vi "Telescope GUI.vi"(9 "Standalone":bool=TRUE, 10 "Init Data":variant, 11 "Telescope Name":string) -> ()   [LabVIEW 2024]
uses:
  typedefs/CC enum Operation Mode.ctl
  Telescope cluster Settings.ctl
  CC cluster Telescope Offsets.ctl
  typedefs/CC cluster sidereal rate.ctl
  Telescope cluster Equinox.ctl
  Telescope cluster Parallax.ctl
  Telescope cluster Rotator.ctl
  Telesope ring Frame.ctl
  Subsystems/SS typedef cluster Instrument Command Queue Data.ctl
  Subsystems/SS cluster Data Queue type.ctl
  Telescope.lvclass
  Telescope cluster Status.ctl
  typedefs/CC cluster RA and DEC.ctl
  Telescope enum Status.ctl
  hk-channel-class/hk-channel-class/HK Item/HK Item.lvclass
  typedefs/CC cluster Object.ctl
  typedefs/cc cluster muRA muDEC.ctl
  typedefs/CC cluster Alarm Data.ctl
  hk-channel-class/hk-channel-class/HK Item/HK Channel cluster Telemetry Data.ctl
  hk-channel-class/hk-channel-class/HK Item/HK Channel enum Data Type.ctl
  hk-channel-class/hk-channel-class/HK Item/HK Item.lvclass/HK Item.ctl
  hk-channel-class/hk-channel-class/HK Alarms/HK Alarm enum Status.ctl
panel:
  in  "Mode":T1
  in  "Tab Control":T2(tab)
  in  "Tab Control 2":T3(tab)
  in  "Target Settings":T4={"RA Proper Motion"=0.0, "DEC Proper Motion"=0.0, "Equinox"=2000.0}
  in  "Wavelength":dbl=1.67
  in  "Frac Rate":dbl=1.0
  in  "Frame":T5=enum."FK5"
  in  "Equinox":T6={"Equinox Year"=2000, "Equinox Prefix"="J"}
  in  "Diff Track":T7
  in  "Parallax":T8
  in  "Rotator":T9={"Frame"="Target", "PA"=0.0}
  in  "Offsets":T10 caption="Offsets (arcSec)"
  in  "Target  DEC Deg":dbl
  in  "Target  RA Deg":dbl
  in  "Target DEC":string
  in  "Target RA":string
  out "DEC Str":string
  out "RA str":string
  out "Moving":bool
  out "Focus Position":dbl format="%.3g"
  out "DEC":dbl
  out "RA":dbl
  out "Telescope Time":timestamp
  out "Connected":bool
  in  "Home Button":bool
  in  "Stop Button":bool
  in  "Move To":bool
  in  "Focus Home":bool
  in  "Move Focus":bool
  in  "Position":dbl format="%.3g"
  in  "Debug":bool
  in  "Reconnect":bool
  in  "Settings Button":bool
  out "Response":string
  in  "Telescope Type":u16(ring) items=["Simulation", "Lowell", "PRIME"]
  out "Messages":string
  out "Cmd Sent":string
  in  "Close":bool
  out "Connect Message":string
  in  "Housekeeping Data":i32(listbox)
  # "Status"
  # "Focus"
  # "HH:MM:SS.s"
  # "Degrees"
  # "HH:MM:SS.s"
  # "Degrees"
  # "microns"
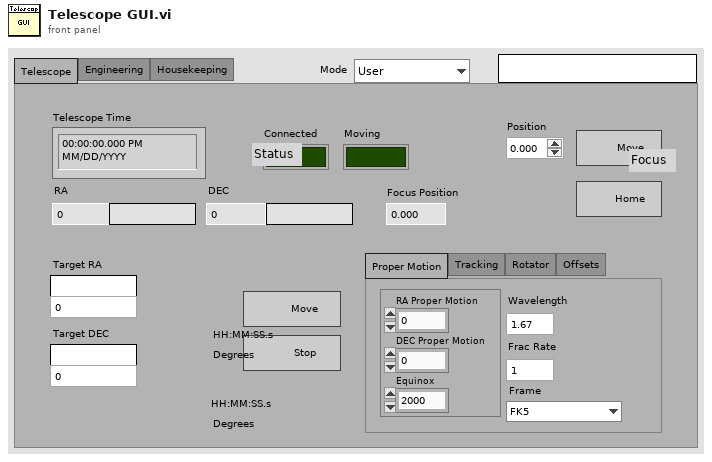
[diagram p1: front panel]
types:
  T1 = typedef "CC enum Operation Mode.ctl" = enum16{"User", "Engineering"}
  T2 = enum32{"Telescope", "Engineering", "Housekeeping"}
  T3 = enum32{"Proper Motion", "Tracking", "Rotator", "Offsets"}
  T4 = typedef "Telescope cluster Settings.ctl" = cluster{"RA Proper Motion":dbl, "DEC Proper Motion":dbl, "Equinox":dbl}
  T5 = typedef "Telesope ring Frame.ctl" = enum16{"FK4", "FK5", "APPT", "GAPPT", "AZEL"}
  T6 = typedef "Telescope cluster Equinox.ctl" = cluster{"Equinox Year":i32, "Equinox Prefix":string}
  T7 = typedef "CC cluster sidereal rate.ctl" = cluster{"dRA":dbl, "dDEC":dbl}
  T8 = typedef "Telescope cluster Parallax.ctl" = cluster{"Parallax":dbl, "rv kps":dbl}
  T9 = typedef "Telescope cluster Rotator.ctl" = cluster{"Frame":string, "PA":dbl}
  T10 = typedef "CC cluster Telescope Offsets.ctl" = cluster{"RA":dbl, "DEC":dbl, "ROT":dbl}
  T11 = typedef "SS typedef cluster Instrument Command Queue Data.ctl" = cluster{"Cmd":string, "Parameters":variant}
  T12 = typedef "Telescope.lvclass/Telescope cluster Status.ctl" = cluster{"Position":T13, "Connected":bool, "Status":T14, "Curr Time":timestamp, "Status Word":u32, "Focus Pos A":dbl, "UTC Time":timestamp, "Local Sidreal Time":dbl, "Azimuth":dbl, "Altitude":dbl, "Rotator Angle":dbl, "RA String":string, "DEC String":string, "secZ":dbl, "Focus Pos B":dbl, "Focus Pos A-B":dbl, "Rotator Offset":dbl, "Time Offset":dbl, "Dome Angle":dbl, "Dome Status Word":u32, "Dome Moving":bool}
  T13 = typedef "CC cluster RA and DEC.ctl" = cluster{"RA":dbl, "DEC":dbl}
  T14 = typedef "Telescope.lvclass/Telescope enum Status.ctl" = enum16{"Initializing", "Ready", "Moving", "Focusing", "Error"}
  T15 = typedef "CC cluster Object.ctl" = cluster{"Object":cluster{"Name":string}, "Sidereal Rate":T7, "RA and DEC":T13, "Proper Motion":T16, "Offsets":T10, "Equinox":T6, "Parallax":T8, "Rotator":T9, "Frame":T5, "Frac Rate":dbl, "Wavelength":dbl}
  T16 = typedef "cc cluster muRA muDEC.ctl" = cluster{"muRA":dbl, "muDEC":dbl, "Epoch":dbl}
  T17 = cluster{"state":refnum<user-event>, "cmd q":refnum<queue>, "Cmd":T11, "Data Q":refnum<queue>, "error":errorcluster, "next poll":timestamp, "Telescope":refnum<class "Telescope.lvclass">, "Telescope Name":string, "poll":bool, "Telescope Status":T12, "Channel List":refnum<class "HK Item.lvclass">[], "Focus Pos":dbl, "Move Position":T15}
  T18 = typedef "CC cluster Alarm Data.ctl" = cluster{"Measured Value":dbl, "Alarm Low":dbl, "Alarm High":dbl, "Message":string, "Source":string}
  T19 = typedef "SS cluster Data Queue type.ctl" = cluster{"Source":string, "Type":string, "Data":variant}
  T20 = enum32{"Page Enabled", "Page Disabled", "Page Disabled & Grayed"}
  T21 = typedef "HK Item.lvclass/HK Channel enum Data Type.ctl" = enum16{"Floating Point", "Integer", "Enum", "String", "Waveform", "File"}
  T22 = typedef "HK Item.lvclass/HK Channel cluster Telemetry Data.ctl" = cluster{"Ch Names":string[], "Ch Values":dbl[], "Timestamp":timestamp, "Data Type":T21}
  T23 = typedef "CC cluster Device Index.ctl" = cluster{"Device Type Name":string, "Curr Device Name":string, "All Instances":string[]}
  T24 = typedef "HK Item.lvclass/HK Channel Units and Setup.ctl" = cluster{"Unit Type":string, "Units":string, "Configuration":string, "Digits":i32, "Data Type":T21, "Exponential?":bool, "Source":string}
  T25 = typedef "HK Item.lvclass/HK Alarm enum Status.ctl" = enum16{"No Alarm", "Red Low", "Red High", "Yellow Low", "Yellow High"}
  T26 = enum32{"invalid app kind", "Development System", "Run Time System", "Student Edition", "Embedded LabVIEW", "Evaluation", "Custom"}
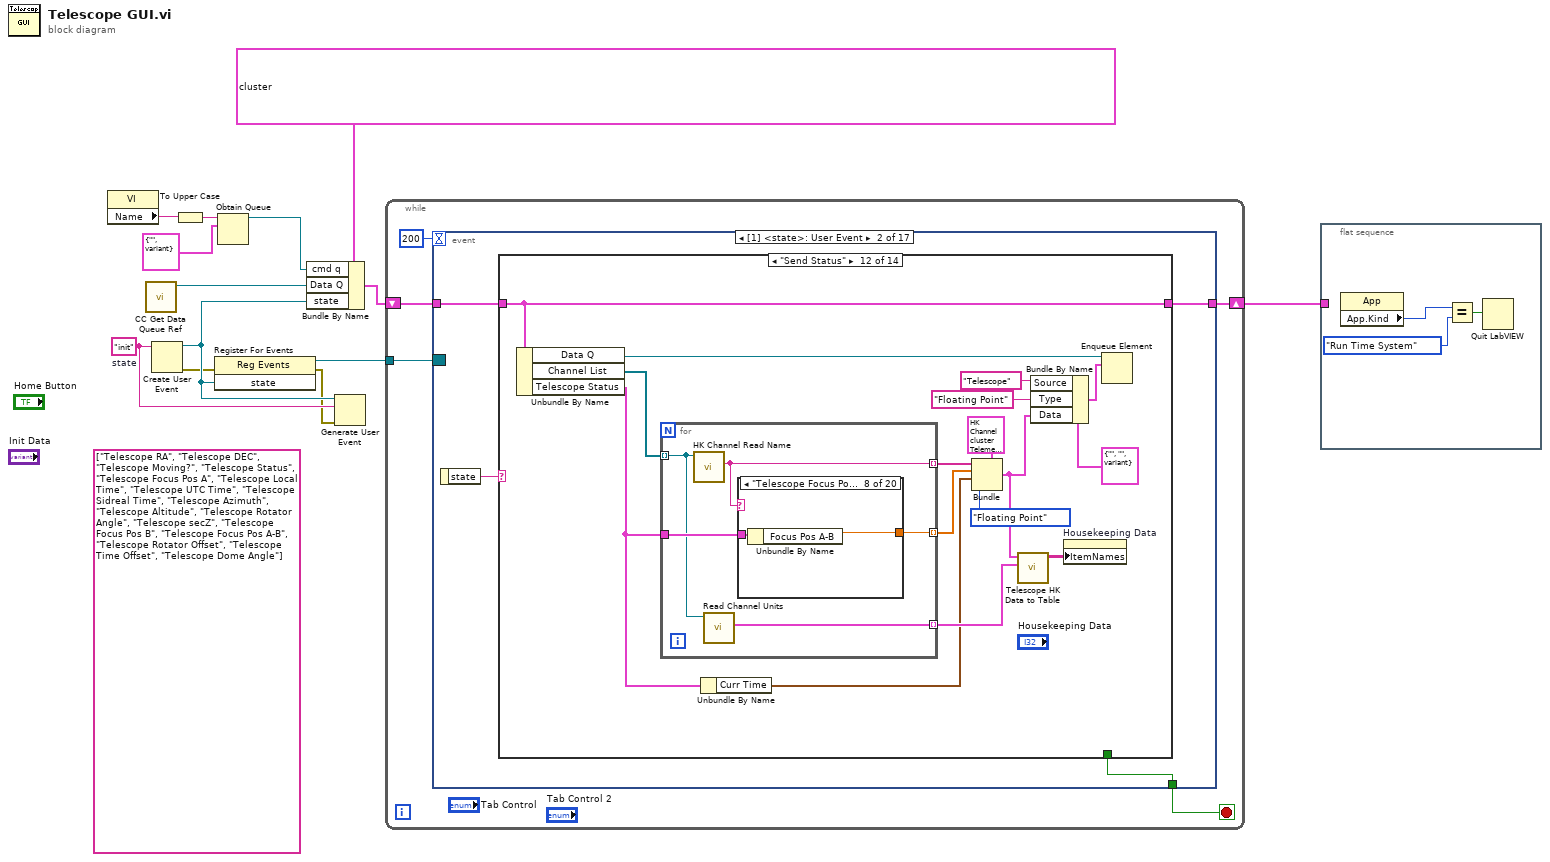
[diagram p0: block diagram]
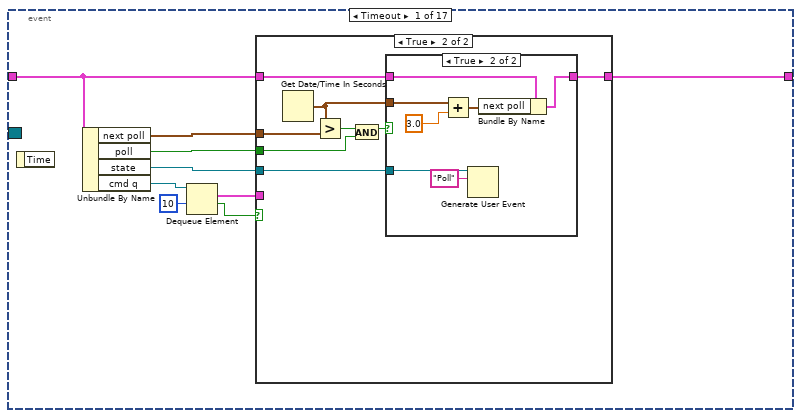
[diagram p2: hidden frame]
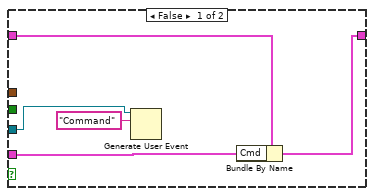
[diagram p3: hidden frame]
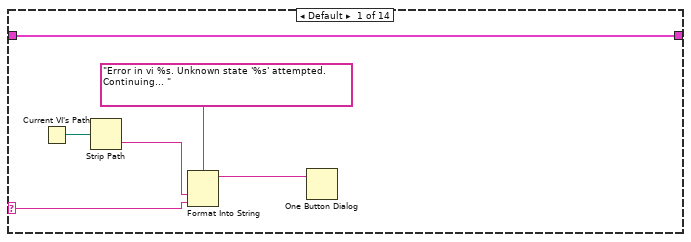
[diagram p5: hidden frame]
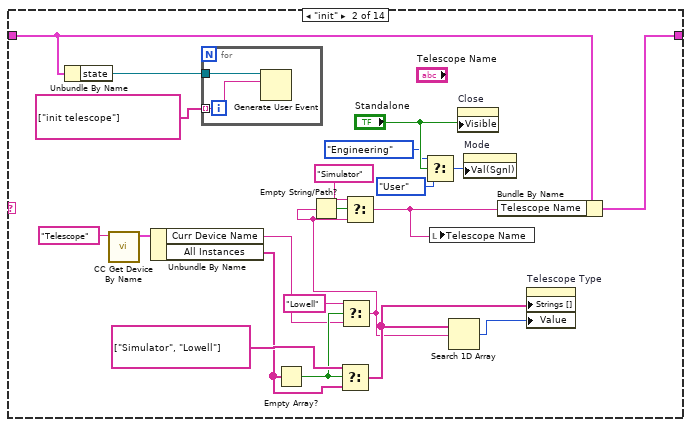
[diagram p6: hidden frame]
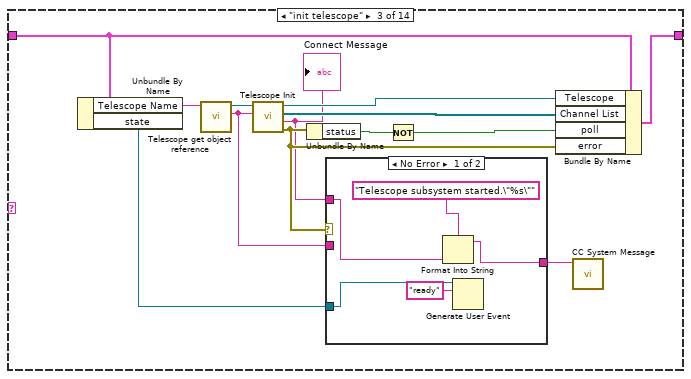
[diagram p7: hidden frame]
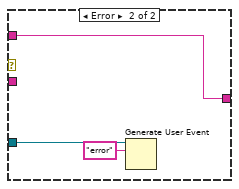
[diagram p8: hidden frame]
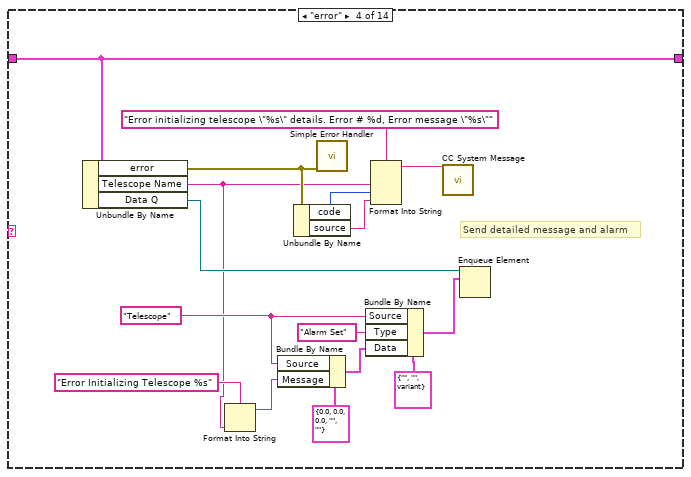
[diagram p9: hidden frame]
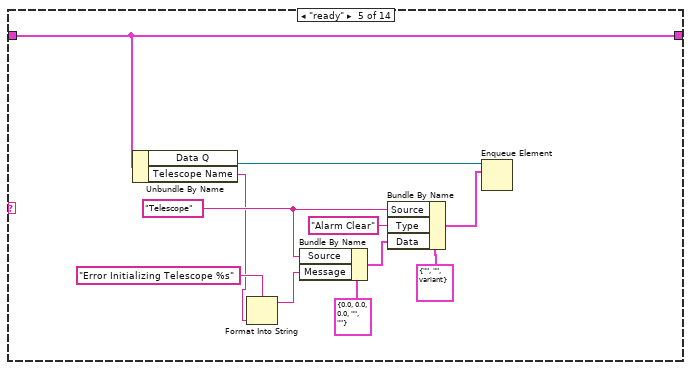
[diagram p10: hidden frame]
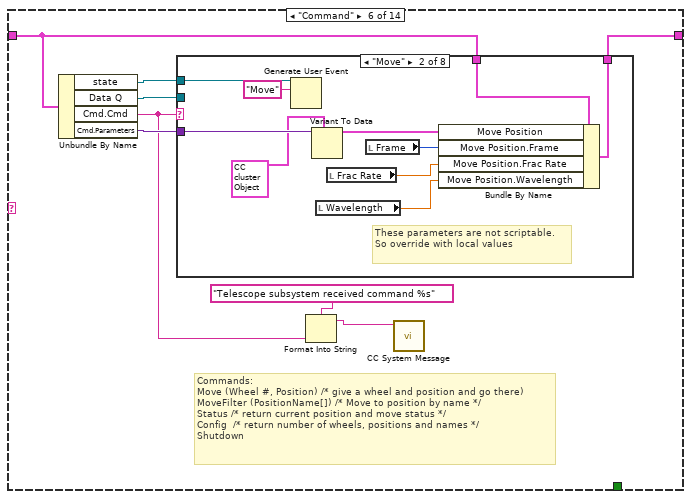
[diagram p11: hidden frame]
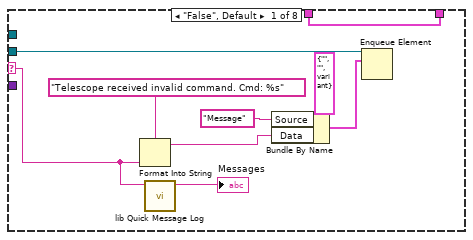
[diagram p12: hidden frame]
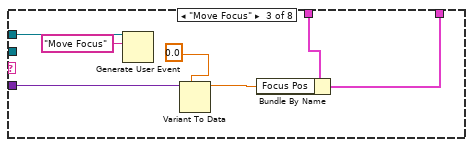
[diagram p13: hidden frame]
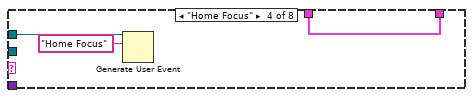
[diagram p14: hidden frame]
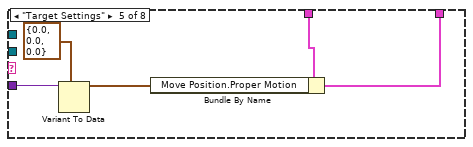
[diagram p15: hidden frame]
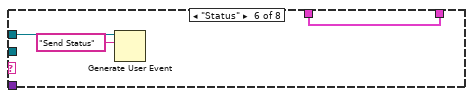
[diagram p16: hidden frame]
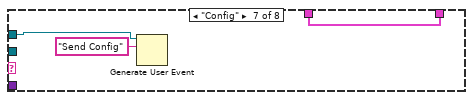
[diagram p17: hidden frame]
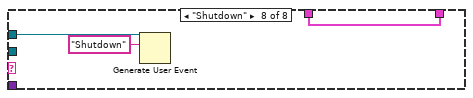
[diagram p18: hidden frame]
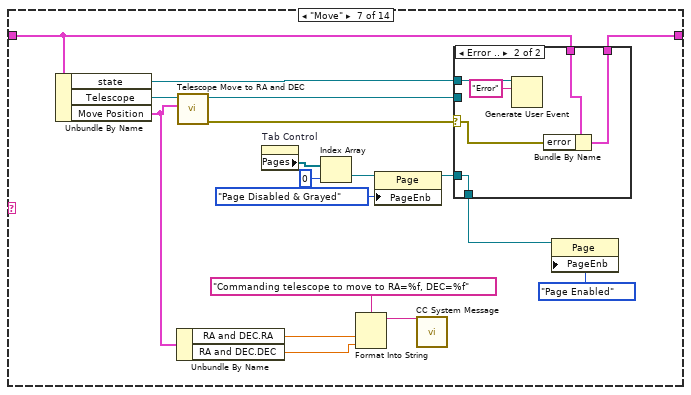
[diagram p19: hidden frame]
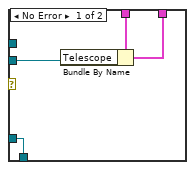
[diagram p20: hidden frame]
diagram:
  (unwired) string[] ["Telescope RA", "Telescope DEC", "Telescope Moving?", "Telescope Status", "Telescope Focus Pos A", "Telescope Local Time", "Telescope UTC Time", "Telescope Sidreal Time", "Telescope Azimuth", "Telescope Altitude", "Telescope Rotator Angle", "Telescope secZ", "Telescope Focus Pos B", "Telescope Focus Pos A-B", "Telescope Rotator Offset", "Telescope Time Offset", "Telescope Dome Angle"]
  w9 = "init"  # state
  n1 = property class="VI"() -> ("Name"=w5:string)  [unwired: 2 in, 2 out]
  n2 = call "CC Get Data Queue Ref.vi"() -> ("Data Q"=w6:refnum<queue>)  [unwired: 10 in, 1 out]
  n3 = Create User Event(user event datatype=w9) -> (user event=w11:refnum<user-event>, error out=w7:errorcluster)  [unwired: 1 in]
  n4 = To Upper Case(1:w5) -> (0:w4:string)
  n5 = register-events(error in=w7, w11) -> (reference out=w10:refnum<event-registration>, error out=w8:errorcluster)  [unwired: 1 in]
  n6 = Obtain Queue(name (unnamed)=w4, element data type=T11 {"Cmd"="", "Parameters"=variant}) -> (queue out=w2:refnum<queue>)  [unwired: 3 in, 2 out]
  n7 = Bundle By Name(cluster=T17 {"state"=refnum, "cmd q"=refnum, "Cmd"={"Cmd"="", "Parameters"=variant}, "Data Q"=refnum, "error"={"status"=FALSE, "code"=0, "source"=""}, "next poll"=timestamp(0 s since 1904-01-01), "Telescope"=refnum, "Telescope Name"="", "poll"=FALSE, "Telescope Status"={"Position"={"RA"=0.0, "DEC"=0.0}, "Connected"=FALSE, "Status"=enum."Initializing", "Curr Time"=timestamp(0 s since 1904-01-01), "Status Word"=0, "Focus Pos A"=0.0, "UTC Time"=timestamp(0 s since 1904-01-01), "Local Sidreal Time"=0.0, "Azimuth"=0.0, "Altitude"=0.0, "Rotator Angle"=0.0, "RA String"="", "DEC String"="", "secZ"=0.0, "Focus Pos B"=0.0, "Focus Pos A-B"=0.0, "Rotator Offset"=0.0, "Time Offset"=0.0, "Dome Angle"=0.0, "Dome Status Word"=0, "Dome Moving"=FALSE}, "Channel List"=[], "Focus Pos"=0.0, "Move Position"={"Object"={"Name"=""}, "Sidereal Rate"={"dRA"=0.0, "dDEC"=0.0}, "RA and DEC"={"RA"=0.0, "DEC"=0.0}, "Proper Motion"={"muRA"=0.0, "muDEC"=0.0, "Epoch"=0.0}, "Offsets"={"RA"=0.0, "DEC"=0.0, "ROT"=0.0}, "Equinox"={"Equinox Year"=0, "Equinox Prefix"=""}, "Parallax"={"Parallax"=0.0, "rv kps"=0.0}, "Rotator"={"Frame"="", "PA"=0.0}, "Frame"=enum."FK4", "Frac Rate"=0.0, "Wavelength"=0.0}}, "cmd q"=w2, "Data Q"=w6, "state"=w11) -> (w12:T17)
  n8 = Generate User Event(user event=w11, event data cluster=w9, error in=w8) -> ()  [unwired: 1 in, 2 out]
  n9 = while {
    tunnel: w10 -> [w18]
    shift-right: [w16] -> w1
    shift-left: w12 -> [w17]
    stop <- w15 stop-if-true
    n10 = event shown="[1] <state>: User Event" {
      selector: w18 -> [_ _ _ _ _ _ _ _ _ _ _ _ _ _ _ _ _]
      dyn-events: _ -> [_ _ _ _ _ _ _ _ _ _ _ _ _ _ _ _ _]
      timeout: 200 -> [_ _ _ _ _ _ _ _ _ _ _ _ _ _ _ _ _]
      tunnel: w17 -> [w22 w51 w366 w367 w376 w398 w401 w404 w409 w414 w417 w420 w424 w430 w437 w441 w448]
      tunnel: [w21 w50 w366 w368 w377 w398 w401 w404 w409 w414 w417 w420 w424 w431 w437 w441 w448] -> w16
      tunnel: [_ w49 _ _ _ _ _ _ _ _ _ _ _ _ _ _ _] -> w15
      event Timeout {
        n11 = event-data() -> ()  [unwired: 1 in, 1 out]
        n12 = Unbundle By Name(w22) -> ("next poll"=w20:timestamp, "poll"=w19:bool, "state"=w23:refnum<user-event>, "cmd q"=w27:refnum<queue>)
        n13 = Dequeue Element(queue=w27, timeout in ms (-1)=10) -> (element=w24:T11, timed out?=w25:bool)  [unwired: 1 in, 2 out]
        n14 = case shown="True" w25 {
          tunnel: w24 -> [w29 _]
          tunnel: w23 -> [w32 w37]
          tunnel: w22 -> [w30 w38]
          tunnel: [w28 w35] -> w21
          tunnel: w20 -> [_ w40]
          tunnel: w19 -> [_ w33]
          frame False {
            n15 = Generate User Event(user event=w32, event data cluster="Command" ("event data")) -> ()  [unwired: 2 in, 2 out]
            n16 = Bundle By Name(cluster=w30, "Cmd"=w29) -> (w28:T17)
          }
          frame True {
            n17 = Get Date/Time In Seconds() -> (seconds since 1Jan1904=w36:timestamp)
            n18 = Greater?(x=w36, y=w40) -> (0:w39:bool)
            n19 = And(x=w39, y=w33) -> (x .and. y?=w34:bool)
            n20 = case shown="True" w34 {
              tunnel: w38 -> [w41 w48]
              tunnel: w37 -> [_ w47]
              tunnel: w36 -> [_ w46]
              tunnel: [w41 w43] -> w35
              frame False {
              }
              frame True {
                n21 = Add(x=w46, y=3.0) -> (x+y=w44:timestamp)
                n22 = Generate User Event(user event=w47, event data cluster="Poll" ("event data")) -> ()  [unwired: 2 in, 2 out]
                n23 = Bundle By Name(cluster=w48, "next poll"=w44) -> (w43:T17)
              }
            }
          }
        }
      }
      event User Event {
        n24 = event-data() -> ("state"=w52:string)  [unwired: 1 in]
        n25 = case shown="\"Send Status\"" w52 {
          selector: w52 -> [w57 _ _ _ _ _ _ _ _ _ _ _ _ _]
          tunnel: w51 -> [w53 w77 w90 w118 w121 w133 w191 w217 w241 w261 w277 w301 w359 w363]
          tunnel: [w53 w78 w91 w118 w121 w134 w192 w218 w242 w261 w278 w301 w359 w363] -> w50
          tunnel: [_ _ _ _ _ _ _ _ _ _ _ _ _ TRUE] -> w49
          frame Default {
            n26 = Current VI's Path() -> (path=w56:path)
            n27 = Strip Path(path=w56) -> (name=w55:string)  [unwired: 1 out]
            n28 = Format Into String(format string="Error in vi %s. Unknown state '%s' attempted. Continuing... ", w55, w57) -> (resulting string=w54:string)  [unwired: 2 in, 1 out]
            n29 = One Button Dialog(message=w54) -> ()  [unwired: 1 in, 1 out]
          }
          frame "init" {
            n30 = Unbundle By Name(w77) -> ("state"=w76:refnum<user-event>)
            n31 = call "CC Get Device By Name.vi"("Device Type"="Telescope") -> ("Device"=w71:T23)  [unwired: 8 in, 2 out]
            n32 = Unbundle By Name(w71) -> ("Curr Device Name"=w61:string, "All Instances"=w63:string[])
            n33 = for {
              tunnel: w76 -> [w81]
              tunnel: string[] ["init telescope"] -> [w80] mode=indexing
              n34 = Generate User Event(user event=w81, event data cluster=w80) -> ()  [unwired: 2 in, 2 out]
            }
            n35 = Empty Array?(array=w63) -> (empty?=w62:bool)
            n36 = Select(t=string[] ["Simulator", "Lowell"] ("All Instances"), s=w62, f=w63) -> (s? t:f=w64:string[])
            n37 = Select(t="Lowell", s=w62, f=w61) -> (s? t:f=w59:string)
            n38 = Empty String/Path?(string/path=w59) -> (empty?=w79:bool)
            n39 = Select(t="Simulator", s=w79, f=w59) -> (s? t:f=w66:string)
            n40 = Select(t=CC_enum_Operation_Mode."Engineering" ("Mode"), s="Standalone", f=CC_enum_Operation_Mode."User" ("Mode")) -> (s? t:f=w67:T1)
            n41 = local write "Telescope Name"(w66) -> ()
            n42 = Search 1D Array(1D array=w64, element=w59) -> (index of element=w74:i32)  [unwired: 1 in]
            n43 = property on="Close" class="Bool"("Visible"="Standalone") -> ()  [unwired: 2 in, 2 out]
            n44 = property on="Mode" class="Enum (strict)"("Val(Sgnl)"=w67) -> ()  [unwired: 2 in, 2 out]
            n45 = Bundle By Name(cluster=w77, "Telescope Name"=w66) -> (w78:T17)
            n46 = property on="Telescope Type" class="Ring (strict)"("Strings []"=w64, "Value"=w74) -> ()  [unwired: 2 in, 2 out]
          }
          frame "init telescope" {
            n47 = Unbundle By Name(w90) -> ("Telescope Name"=w93:string, "state"=w84:refnum<user-event>)
            n48 = call "Telescope get object reference.vi"("Telescope Name"=w93) -> ("Telescope Name dup"=w85:string, "PRIME Telescope.lvclass"=w94:refnum<class "Telescope.lvclass">)  [unwired: 8 in, 1 out]
            n49 = call-dynamic "Telescope Init.vi"("Name"=w85, "Telescope in"=w94) -> ("error out"=w83:errorcluster, "Connect Message"=w82:string, "Channel List"=w87:refnum<class "HK Item.lvclass">[], "Telescope out"=w92:refnum<class "Telescope.lvclass">)  [unwired: 6 in]
            "Connect Message" <- w82
            n50 = Unbundle By Name(w83) -> ("status"=w89:bool)
            n51 = case shown="No Error" w83 {
              tunnel: [w99 w100] -> w86
              tunnel: w85 -> [_ _]
              tunnel: w84 -> [w96 w102]
              tunnel: w82 -> [w97 w100]
              frame No Error {
                n52 = Format Into String(format string="Telescope subsystem started.\"%s\"", w97) -> (resulting string=w99:string)  [unwired: 2 in, 1 out]
                n53 = Generate User Event(user event=w96, event data cluster="ready" ("event data")) -> ()  [unwired: 2 in, 2 out]
              }
              frame Error {
                n54 = Generate User Event(user event=w102, event data cluster="error" ("event data")) -> ()  [unwired: 2 in, 2 out]
              }
            }
            n55 = Not(x=w89) -> (.not. x?=w88:bool)
            n56 = Bundle By Name(cluster=w90, "Telescope"=w92, "Channel List"=w87, "poll"=w88, "error"=w83) -> (w91:T17)
            n57 = call "CC System Message.vi"("Message"=w86) -> ()  [unwired: 10 in, 1 out]
          }
          frame "error" {
            w113 = "Telescope" ("Source")
            # "Send detailed message and alarm"
            n58 = Unbundle By Name(w118) -> ("error"=w110:errorcluster, "Telescope Name"=w103:string, "Data Q"=w107:refnum<queue>)
            n59 = Format Into String(format string="Error Initializing Telescope %s" ("Message"), w103) -> (resulting string=w104:string)  [unwired: 2 in, 1 out]
            n60 = Bundle By Name(cluster=T18 {"Measured Value"=0.0, "Alarm Low"=0.0, "Alarm High"=0.0, "Message"="", "Source"=""} ("element"), "Source"=w113, "Message"=w104) -> (w114:T18)
            n61 = Unbundle By Name(w110) -> ("code"=w112:i32, "source"=w111:string)
            n62 = call <vilib>:"Simple Error Handler.vi"("error in (no error)"=w110) -> ()  [unwired: 4 in, 5 out]
            n63 = Bundle By Name(cluster=T19 {"Source"="", "Type"="", "Data"=variant} ("element"), "Source"=w113, "Type"="Alarm Set", "Data"=w114) -> (w106:T19)
            n64 = Format Into String(format string="Error initializing telescope \"%s\" details. Error # %d, Error message \"%s\"", w103, w112, w111) -> (resulting string=w109:string)  [unwired: 2 in, 1 out]
            n65 = call "CC System Message.vi"("Message"=w109) -> ()  [unwired: 10 in, 1 out]
            n66 = Enqueue Element(queue=w107, element=w106) -> ()  [unwired: 2 in, 3 out]
          }
          frame "ready" {
            w125 = "Telescope" ("Source")
            n67 = Unbundle By Name(w121) -> ("Data Q"=w120:refnum<queue>, "Telescope Name"=w119:string)
            n68 = Format Into String(format string="Error Initializing Telescope %s" ("Message"), w119) -> (resulting string=w122:string)  [unwired: 2 in, 1 out]
            n69 = Bundle By Name(cluster=T18 {"Measured Value"=0.0, "Alarm Low"=0.0, "Alarm High"=0.0, "Message"="", "Source"=""} ("element"), "Source"=w125, "Message"=w122) -> (w126:T18)
            n70 = Bundle By Name(cluster=T19 {"Source"="", "Type"="", "Data"=variant} ("element"), "Source"=w125, "Type"="Alarm Clear", "Data"=w126) -> (w124:T19)
            n71 = Enqueue Element(queue=w120, element=w124) -> ()  [unwired: 2 in, 3 out]
          }
          frame "Command" {
            # "Commands:\nMove (Wheel #, Position) /* give a wheel and position and go there)\nMoveFilter (PositionName[]) /* Move to position by name */\nStatus /* return current position and move status */\nConfig  /* return number of wheels, positions and names */\nShutdown"
            n72 = Unbundle By Name(w133) -> ("state"=w135:refnum<user-event>, "Data Q"=w137:refnum<queue>, "Cmd.Cmd"=w131:string, "Cmd.Parameters"=w136:variant)
            n73 = case shown="\"Move\"" w131 {
              selector: w131 -> [w140 _ _ _ _ _ _ _]
              tunnel: w137 -> [w146 _ _ _ _ _ _ _]
              tunnel: w136 -> [_ w156 w163 _ w171 _ _ _]
              tunnel: w135 -> [_ w152 w159 w166 _ w174 w176 w180]
              tunnel: w133 -> [w138 w155 w162 w164 w169 w172 w175 w178]
              tunnel: [w138 w153 w160 w164 w167 w172 w175 w178] -> w134
              frame "False", Default {
                n74 = Format Into String(format string="Telescope received invalid command. Cmd: %s", w140) -> (resulting string=w142:string)  [unwired: 2 in, 1 out]
                n75 = call "lib Quick Message Log.vi"("Message"=w140) -> ("Log"=→"Messages":string)  [unwired: 9 in, 1 out]
                n76 = Bundle By Name(cluster=T19 {"Source"="", "Type"="", "Data"=variant} ("element"), "Source"="Message" ("Data Type"), "Data"=w142) -> (w141:T19)
                n77 = Enqueue Element(queue=w146, element=w141) -> ()  [unwired: 2 in, 3 out]
              }
              frame "Move" {
                # "These parameters are not scriptable. So override with local values"
                n78 = Generate User Event(user event=w152, event data cluster="Move" ("event data")) -> ()  [unwired: 2 in, 2 out]
                n79 = Variant To Data(type=T15 {"Object"={"Name"=""}, "Sidereal Rate"={"dRA"=0.0, "dDEC"=0.0}, "RA and DEC"={"RA"=0.0, "DEC"=0.0}, "Proper Motion"={"muRA"=0.0, "muDEC"=0.0, "Epoch"=0.0}, "Offsets"={"RA"=0.0, "DEC"=0.0, "ROT"=0.0}, "Equinox"={"Equinox Year"=0, "Equinox Prefix"=""}, "Parallax"={"Parallax"=0.0, "rv kps"=0.0}, "Rotator"={"Frame"="", "PA"=0.0}, "Frame"=enum."FK4", "Frac Rate"=0.0, "Wavelength"=0.0} ("Move Position"), Variant=w156) -> (data=w154:T15)  [unwired: 1 in, 1 out]
                n80 = local read "Wavelength"() -> (w147:dbl)
                n81 = local read "Frac Rate"() -> (w148:dbl)
                n82 = local read "Frame"() -> (w149:T5)
                n83 = Bundle By Name(cluster=w155, "Move Position"=w154, "Move Position.Frame"=w149, "Move Position.Frac Rate"=w148, "Move Position.Wavelength"=w147) -> (w153:T17)
              }
              frame "Move Focus" {
                n84 = Generate User Event(user event=w159, event data cluster="Move Focus" ("event data")) -> ()  [unwired: 2 in, 2 out]
                n85 = Variant To Data(type=0.0 ("Position"), Variant=w163) -> (data=w161:dbl)  [unwired: 1 in, 1 out]
                n86 = Bundle By Name(cluster=w162, "Focus Pos"=w161) -> (w160:T17)
              }
              frame "Home Focus" {
                n87 = Generate User Event(user event=w166, event data cluster="Home Focus" ("event data")) -> ()  [unwired: 2 in, 2 out]
              }
              frame "Target Settings" {
                n88 = Variant To Data(type=T4 {"RA Proper Motion"=0.0, "DEC Proper Motion"=0.0, "Equinox"=0.0} ("Telescope Settings"), Variant=w171) -> (data=w168:T4)  [unwired: 1 in, 1 out]
                n89 = Bundle By Name(cluster=w169, "Move Position.Proper Motion"=w168) -> (w167:T17)
              }
              frame "Status" {
                n90 = Generate User Event(user event=w174, event data cluster="Send Status" ("event data")) -> ()  [unwired: 2 in, 2 out]
              }
              frame "Config" {
                n91 = Generate User Event(user event=w176, event data cluster="Send Config" ("event data")) -> ()  [unwired: 2 in, 2 out]
              }
              frame "Shutdown" {
                n92 = Generate User Event(user event=w180, event data cluster="Shutdown" ("event data")) -> ()  [unwired: 2 in, 2 out]
              }
            }
            n93 = Format Into String(format string="Telescope subsystem received command %s", w131) -> (resulting string=w130:string)  [unwired: 2 in, 1 out]
            n94 = call "CC System Message.vi"("Message"=w130) -> ()  [unwired: 10 in, 1 out]
          }
          frame "Move" {
            n95 = Unbundle By Name(w191) -> ("state"=w193:refnum<user-event>, "Telescope"=w188:refnum<class "Telescope.lvclass">, "Move Position"=w181:T15)
            n96 = Unbundle By Name(w181) -> ("RA and DEC.RA"=w183:dbl, "RA and DEC.DEC"=w182:dbl)
            n97 = call-dynamic "Telescope Move to RA and DEC.vi"("Object out"=w181, "Telescope in"=w188) -> ("error out"=w187:errorcluster, "Telescope out"=w186:refnum<class "Telescope.lvclass">)  [unwired: 8 in]
            n98 = property on="Tab Control" class="TabCtl (strict)"() -> ("Pages"=w198:refnum<vi>[])  [unwired: 2 in, 2 out]
            n99 = Index Array(array=w198, index=0) -> (element=w196:refnum<vi>)
            n100 = Format Into String(format string="Commanding telescope to move to RA=%f, DEC=%f", w183, w182) -> (resulting string=w184:string)  [unwired: 2 in, 1 out]
            n101 = property class="Page"(reference=w196, "PageEnb"=T20."Page Disabled & Grayed" ("Page Enabled State")) -> (reference out=w190:refnum<vi>)  [unwired: 1 in, 1 out]
            n102 = call "CC System Message.vi"("Message"=w184) -> ()  [unwired: 10 in, 1 out]
            n103 = case shown="Error .." w187 {
              selector: w187 -> [_ w205]
              tunnel: w193 -> [_ w208]
              tunnel: w191 -> [w201 w206]
              tunnel: [w199 w204] -> w192
              tunnel: w190 -> [w202 w203]
              tunnel: [w202 w203] -> w189
              tunnel: w186 -> [w200 _]
              frame No Error {
                n104 = Bundle By Name(cluster=w201, "Telescope"=w200) -> (w199:T17)
              }
              frame Error {
                n105 = Generate User Event(user event=w208, event data cluster="Error" ("event data")) -> ()  [unwired: 2 in, 2 out]
                n106 = Bundle By Name(cluster=w206, "error"=w205) -> (w204:T17)
              }
            }
            n107 = property class="Page"(reference=w189, "PageEnb"=T20."Page Enabled" ("Page Enabled State")) -> ()  [unwired: 1 in, 2 out]
          }
          frame "Move Focus" {
            n108 = Unbundle By Name(w217) -> ("state"=w219:refnum<user-event>, "Telescope"=w214:refnum<class "Telescope.lvclass">, "Focus Pos"=w210:dbl)
            n109 = call-dynamic "Telescope Move Focus.vi"("Focus Pos"=w210, "Telescope in"=w214) -> ("error out"=w213:errorcluster, "Telescope out"=w212:refnum<class "Telescope.lvclass">)  [unwired: 8 in]
            n110 = property on="Tab Control" class="TabCtl (strict)"() -> ("Pages"=w224:refnum<vi>[])  [unwired: 2 in, 2 out]
            n111 = Index Array(array=w224, index=0) -> (element=w222:refnum<vi>)
            n112 = Format Into String(format string="Commanding telescope to move focus to position %f", w210) -> (resulting string=w211:string)  [unwired: 2 in, 1 out]
            n113 = property class="Page"(reference=w222, "PageEnb"=T20."Page Disabled & Grayed" ("Page Enabled State")) -> (reference out=w216:refnum<vi>)  [unwired: 1 in, 1 out]
            n114 = call "CC System Message.vi"("Message"=w211) -> ()  [unwired: 10 in, 1 out]
            n115 = case shown="No Error" w213 {
              selector: w213 -> [_ w231]
              tunnel: w219 -> [_ w234]
              tunnel: w217 -> [w227 w232]
              tunnel: [w225 w230] -> w218
              tunnel: w216 -> [w228 w229]
              tunnel: [w228 w229] -> w215
              tunnel: w212 -> [w226 _]
              frame No Error {
                n116 = Bundle By Name(cluster=w227, "Telescope"=w226) -> (w225:T17)
              }
              frame Error {
                n117 = Generate User Event(user event=w234, event data cluster="Error" ("event data")) -> ()  [unwired: 2 in, 2 out]
                n118 = Bundle By Name(cluster=w232, "error"=w231) -> (w230:T17)
              }
            }
            n119 = property class="Page"(reference=w215, "PageEnb"=T20."Page Enabled" ("Page Enabled State")) -> ()  [unwired: 1 in, 2 out]
          }
          frame "Home Focus" {
            n120 = Unbundle By Name(w241) -> ("state"=w243:refnum<user-event>, "Telescope"=w238:refnum<class "Telescope.lvclass">)
            n121 = call-dynamic "Telescope Home Focus.vi"("Telescope in"=w238) -> ("error out"=w237:errorcluster, "Telescope out"=w236:refnum<class "Telescope.lvclass">)  [unwired: 9 in]
            n122 = property on="Tab Control" class="TabCtl (strict)"() -> ("Pages"=w248:refnum<vi>[])  [unwired: 2 in, 2 out]
            n123 = Index Array(array=w248, index=0) -> (element=w246:refnum<vi>)
            n124 = property class="Page"(reference=w246, "PageEnb"=T20."Page Disabled & Grayed" ("Page Enabled State")) -> (reference out=w240:refnum<vi>)  [unwired: 1 in, 1 out]
            n125 = call "CC System Message.vi"("Message"="Commanding telescope to move focus to home position" ("format string")) -> ()  [unwired: 10 in, 1 out]
            n126 = case shown="Error .." w237 {
              selector: w237 -> [_ w255]
              tunnel: w243 -> [_ w258]
              tunnel: w241 -> [w251 w256]
              tunnel: [w249 w254] -> w242
              tunnel: w240 -> [w252 w253]
              tunnel: [w252 w253] -> w239
              tunnel: w236 -> [w250 _]
              frame No Error {
                n127 = Bundle By Name(cluster=w251, "Telescope"=w250) -> (w249:T17)
              }
              frame Error {
                n128 = Generate User Event(user event=w258, event data cluster="Error" ("event data")) -> ()  [unwired: 2 in, 2 out]
                n129 = Bundle By Name(cluster=w256, "error"=w255) -> (w254:T17)
              }
            }
            n130 = property class="Page"(reference=w239, "PageEnb"=T20."Page Enabled" ("Page Enabled State")) -> ()  [unwired: 1 in, 2 out]
          }
          frame "Stop" {
            n131 = Unbundle By Name(w261) -> ("Telescope"=w260:refnum<class "Telescope.lvclass">)
            n132 = call-dynamic "Telescope Stop.vi"("Telescope in"=w260) -> ()  [unwired: 9 in, 2 out]
            n133 = call "CC System Message.vi"("Message"="Commanding telescope to stop all motion.") -> ()  [unwired: 10 in, 1 out]
          }
          frame "Poll" {
            # "Request status from hardware"
            n134 = Unbundle By Name(w277) -> ("Telescope"=w280:refnum<class "Telescope.lvclass">, "state"=w271:refnum<user-event>)
            n135 = Generate User Event(user event=w271, event data cluster="Send Status" ("event data")) -> ()  [unwired: 2 in, 2 out]
            n136 = call-dynamic "Telescope Read Current Status.vi"("Telescope in"=w280) -> ("Raw Response"=→"Response":string, "Telescope Status"=w276:T12, "Telescope out"=w279:refnum<class "Telescope.lvclass">, "Cmd Sent"=→"Cmd Sent":string)  [unwired: 6 in, 1 out]
            n137 = Unbundle By Name(w276) -> ("Position.RA"=w266:dbl, "Position.DEC"=w265:dbl, "Curr Time"=→"Telescope Time":timestamp, "Connected"=→"Connected":bool, "Focus Pos A"=→"Focus Position":dbl, "Status"=w268:T14)
            "RA" <- w266
            "DEC" <- w265
            n138 = Bundle By Name(cluster=w277, "Telescope"=w279, "Telescope Status"=w276) -> (w278:T17)
            n139 = case shown="\"Focusing\"" w268 {
              tunnel: [FALSE FALSE TRUE TRUE FALSE] -> w267
              frame "Initializing", Default {
              }
              frame "Ready" {
              }
              frame "Moving" {
              }
              frame "Focusing" {
              }
              frame "Error" {
              }
            }
            "Moving" <- w267
            n140 = Bundle("RA"=w266, "DEC"=w265) -> (w264:cluster{"RA":dbl, "DEC":dbl})  [unwired: 1 in]
            n141 = call "Telescope Convert RA and DEC to HHMMSS.vi"("RA and DEC"=w264) -> ("Dec String"=→"DEC Str":string, "RA String"=→"RA str":string)  [unwired: 7 in, 2 out]
          }
          frame "Send Status" {
            n142 = Unbundle By Name(w301) -> ("Data Q"=w300:refnum<queue>, "Channel List"=w295:refnum<class "HK Item.lvclass">[], "Telescope Status"=w292:T12)
            n143 = for {
              tunnel: w295 -> [w305] mode=indexing
              tunnel: w292 -> [w306]
              tunnel: [w303] -> w293 mode=indexing
              tunnel: [w304] -> w294 mode=indexing
              tunnel: [w302] -> w289 mode=indexing
              n144 = call "HK Channel Read Name.vi"("HK Item in"=w305) -> ("Name"=w304:string)  [unwired: 8 in, 2 out]
              n145 = call "Read Channel Units.vi"("HK Item in"=w305) -> ("Channel Setup"=w302:T24)  [unwired: 8 in, 2 out]
              n146 = case shown="\"Telescope Focus Pos A-B\"" w304 {
                tunnel: w306 -> [_ w309 w311 w319 w321 w323 w325 w327 w330 w333 w335 w337 w339 w341 w343 w345 w347 w349 w351 w354]
                tunnel: [nan ("DEC") w308 w310 w317 w320 w322 w324 w326 w328 w331 w334 w336 w338 w340 w342 w344 w346 w348 w350 w352] -> w303
                frame "False", Default {
                  (unwired) HK_Alarm_enum_Status."No Alarm" ("Alarm Status")
                }
                frame "Telescope RA" {
                  n147 = Unbundle By Name(w309) -> ("Position.RA"=w308:dbl)
                }
                frame "Telescope DEC" {
                  n148 = Unbundle By Name(w311) -> ("Position.DEC"=w310:dbl)
                }
                frame "Telescope Moving?" {
                  n149 = Unbundle By Name(w319) -> ("Status"=w315:T14)
                  n150 = Equal?(x=w315, y=Telescope_enum_Status."Moving") -> (x = y?=w316:bool)
                  n151 = Equal?(x=Telescope_enum_Status."Focusing" ("y"), y=w315) -> (x = y?=w313:bool)
                  n152 = Or(x=w313, y=w316) -> (x .or. y?=w314:bool)
                  n153 = Boolean To (0,1)(Boolean=w314) -> (0, 1=w317:i16)
                }
                frame "Telescope Status" {
                  n154 = Unbundle By Name(w321) -> ("Status Word"=w320:u32)
                }
                frame "Telescope Focus Pos A" {
                  n155 = Unbundle By Name(w323) -> ("Focus Pos A"=w322:dbl)
                }
                frame "Telescope Focus Pos B" {
                  n156 = Unbundle By Name(w325) -> ("Focus Pos B"=w324:dbl)
                }
                frame "Telescope Focus Pos A-B" {
                  n157 = Unbundle By Name(w327) -> ("Focus Pos A-B"=w326:dbl)
                }
                frame "Telescope Local Time" {
                  n158 = Unbundle By Name(w330) -> ("Curr Time"=w329:timestamp)
                  n159 = To Double Precision Float(number=w329) -> (double precision float=w328:dbl)
                }
                frame "Telescope UTC Time" {
                  n160 = Unbundle By Name(w333) -> ("UTC Time"=w332:timestamp)
                  n161 = To Double Precision Float(number=w332) -> (double precision float=w331:dbl)
                }
                frame "Telescope Sidreal Time" {
                  n162 = Unbundle By Name(w335) -> ("Local Sidreal Time"=w334:dbl)
                }
                frame "Telescope Azimuth" {
                  n163 = Unbundle By Name(w337) -> ("Azimuth"=w336:dbl)
                }
                frame "Telescope Elevation" {
                  n164 = Unbundle By Name(w339) -> ("Altitude"=w338:dbl)
                }
                frame "Telescope Rotator Angle" {
                  n165 = Unbundle By Name(w341) -> ("Rotator Angle"=w340:dbl)
                }
                frame "Telescope secZ" {
                  n166 = Unbundle By Name(w343) -> ("secZ"=w342:dbl)
                }
                frame "Telescope Rotator Offset" {
                  n167 = Unbundle By Name(w345) -> ("Rotator Offset"=w344:dbl)
                }
                frame "Telescope Time Offset" {
                  n168 = Unbundle By Name(w347) -> ("Time Offset"=w346:dbl)
                }
                frame "Telescope Dome Angle" {
                  n169 = Unbundle By Name(w349) -> ("Dome Angle"=w348:dbl)
                }
                frame "Telescope Dome Status" {
                  n170 = Unbundle By Name(w351) -> ("Dome Status Word"=w350:u32)
                }
                frame "Telescope Dome Moving?" {
                  n171 = Unbundle By Name(w354) -> ("Dome Moving"=w353:bool)
                  n172 = Boolean To (0,1)(Boolean=w353) -> (0, 1=w352:i16)
                }
              }
            }
            n173 = Unbundle By Name(w292) -> ("Curr Time"=w287:timestamp)
            n174 = Bundle(cluster=T22 {"Ch Names"=[], "Ch Values"=[], "Timestamp"=timestamp(0 s since 1904-01-01), "Data Type"=enum."Floating Point"}, "Ch Names"=w294, "Ch Values"=w293, "Timestamp"=w287, "Data Type"=HK_Channel_enum_Data_Type."Floating Point") -> (w290:T22)
            n175 = call "Telescope HK Data to Table.vi"("Ch Info"=w289, "HK Data Cluster"=w290) -> ("Table"=w288:string[][])  [unwired: 9 in]
            n176 = Bundle By Name(cluster=T19 {"Source"="", "Type"="", "Data"=variant} ("element"), "Source"="Telescope", "Type"="Floating Point" ("Data Type"), "Data"=w290) -> (w297:T19)
            n177 = property on="Housekeeping Data" class="MCListbox (strict)"("ItemNames"=w288) -> ()  [unwired: 2 in, 2 out]
            n178 = Enqueue Element(queue=w300, element=w297) -> ()  [unwired: 2 in, 3 out]
          }
          frame "Reinit" {
            n179 = Unbundle By Name(w359) -> ("Telescope"=w358:refnum<class "Telescope.lvclass">, "state"=w357:refnum<user-event>)
            n180 = call-dynamic "Telescope Close.vi"("Telescope in"=w358) -> ("error out"=w355:errorcluster)  [unwired: 9 in, 1 out]
            n181 = Generate User Event(user event=w357, event data cluster="init telescope" ("event data")) -> ()  [unwired: 2 in, 2 out]
            n182 = call <vilib>:"Clear Errors.vi"("error in (no error)"=w355) -> ()  [unwired: 5 in, 2 out]
          }
          frame "Shutdown" {
            n183 = Unbundle By Name(w363) -> ("Data Q"=w362:refnum<queue>, "Telescope"=w360:refnum<class "Telescope.lvclass">)
            n184 = Release Queue(queue=w362) -> ()  [unwired: 2 in, 3 out]
            n185 = call-dynamic "Telescope Close.vi"("Telescope in"=w360) -> ()  [unwired: 9 in, 2 out]
            n186 = call "CC System Message.vi"("Message"="Telescope shutdown.") -> ()  [unwired: 10 in, 1 out]
          }
        }
      }
      event "Standalone": Value Change {
        n187 = event-data() -> ("NewVal"=w365:bool)  [unwired: 1 in, 5 out]
        n188 = property on="Close" class="Bool"("Visible"=w365) -> ()  [unwired: 2 in, 2 out]
      }
      event "Debug": Value Change {
        n189 = event-data() -> ()  [unwired: 1 in, 6 out]
        n190 = Unbundle By Name(w367) -> ("Telescope"=w371:refnum<class "Telescope.lvclass">)
        n191 = call-dynamic "Telescope Debug.vi"("Debug"="Debug", "Telescope in"=w371) -> ("Telescope out"=w369:refnum<class "Telescope.lvclass">)  [unwired: 8 in, 1 out]
        n192 = Bundle By Name(cluster=w367, "Telescope"=w369) -> (w368:T17)
      }
      event "Settings Button": Value Change {
        n193 = event-data() -> ()  [unwired: 1 in, 6 out]
        n194 = Unbundle By Name(w376) -> ("Telescope"=w379:refnum<class "Telescope.lvclass">, "Telescope Name"=w372:string, "state"=w374:refnum<user-event>)
        n195 = call-dynamic "Telescope Configure GUI.vi"("Telescope Name"=w372, "Telescope in"=w379) -> ("Telescope out"=w378:refnum<class "Telescope.lvclass">)  [unwired: 8 in, 1 out]
        n196 = Generate User Event(user event=w374, event data cluster="Reinit" ("event data")) -> ()  [unwired: 2 in, 2 out]
        n197 = Bundle By Name(cluster=w376, "Telescope"=w378) -> (w377:T17)
        n198 = call "CC System Message.vi"("Message"="Telescope settings updated.") -> ()  [unwired: 10 in, 1 out]
      }
      event "Move To": Value Change {
        n199 = event-data() -> ()  [unwired: 1 in, 1 out]
        n200 = Unbundle By Name(w398) -> ("cmd q"=w393:refnum<queue>, "Move Position"=w392:T15)
        n201 = call "Telescope Convert HHMMSS to RA and DEC Angle.vi"("Dec String"="Target DEC", "RA String"="Target RA") -> ("RA and DEC"=w390:T13)  [unwired: 7 in, 2 out]
        n202 = Bundle By Name(cluster=w392, "Object.Name"="Telescope Manual Move", "Proper Motion"="Target Settings", "Offsets"="Offsets", "RA and DEC"=w390, "Parallax"="Parallax", "Rotator"="Rotator", "Frame"="Frame", "Frac Rate"="Frac Rate", "Wavelength"="Wavelength", "Equinox"="Equinox", "Sidereal Rate"="Diff Track") -> (w391:T15)
        n203 = Bundle By Name(cluster=T11 {"Cmd"="Move", "Parameters"=variant} ("element"), "Parameters"=w391) -> (w396:T11)
        n204 = Enqueue Element(queue=w393, element=w396) -> ()  [unwired: 2 in, 3 out]
      }
      event "Target RA": Value Change {
        n205 = event-data() -> ("NewVal"=w400:string)  [unwired: 1 in]
        n206 = call "Telescope Convert HHMMSS to RA and DEC Angle.vi"("RA String"=w400) -> ("RA"=w399:dbl)  [unwired: 8 in, 2 out]
        n207 = local write "Target  RA Deg"(w399) -> ()
      }
      event "Target DEC": Value Change {
        n208 = event-data() -> ("NewVal"=w403:string)  [unwired: 1 in]
        n209 = call "Telescope Convert HHMMSS to RA and DEC Angle.vi"("Dec String"=w403) -> ("DEC"=w402:dbl)  [unwired: 8 in, 2 out]
        n210 = local write "Target  DEC Deg"(w402) -> ()
      }
      event "Target  RA Deg": Value Change {
        n211 = event-data() -> ()  [unwired: 1 in, 6 out]
        n212 = Bundle By Name(cluster=T13 {"RA"=0.0, "DEC"=0.0} ("RA and DEC"), "RA"="Target  RA Deg") -> (w406:T13)
        n213 = call "Telescope Convert RA and DEC to HHMMSS.vi"("RA and DEC"=w406) -> ("RA String"=w405:string)  [unwired: 7 in, 3 out]
        n214 = local write "Target RA"(w405) -> ()
      }
      event "Target  DEC Deg": Value Change {
        n215 = event-data() -> ()  [unwired: 1 in, 6 out]
        n216 = Bundle By Name(cluster=T13 {"RA"=0.0, "DEC"=0.0} ("RA and DEC"), "DEC"="Target  DEC Deg") -> (w412:T13)
        n217 = call "Telescope Convert RA and DEC to HHMMSS.vi"("RA and DEC"=w412) -> ("Dec String"=w410:string)  [unwired: 7 in, 3 out]
        n218 = local write "Target DEC"(w410) -> ()
      }
      event "Stop Button": Value Change {
        n219 = event-data() -> ()  [unwired: 1 in, 6 out]
        n220 = Unbundle By Name(w417) -> ("state"=w416:refnum<user-event>)
        n221 = Generate User Event(user event=w416, event data cluster="Stop" ("event data")) -> ()  [unwired: 2 in, 2 out]
      }
      event "Move Focus": Value Change {
        n222 = event-data() -> ()  [unwired: 1 in, 6 out]
        n223 = Unbundle By Name(w420) -> ("cmd q"=w422:refnum<queue>)
        n224 = Bundle By Name(cluster=T11 {"Cmd"="Move Focus", "Parameters"=variant} ("element"), "Parameters"="Position") -> (w418:T11)
        n225 = Enqueue Element(queue=w422, element=w418) -> ()  [unwired: 2 in, 3 out]
      }
      event "Focus Home": Value Change {
        n226 = event-data() -> ()  [unwired: 1 in, 6 out]
        n227 = Unbundle By Name(w424) -> ("cmd q"=w425:refnum<queue>)
        n228 = Enqueue Element(queue=w425, element=T11 {"Cmd"="Home Focus", "Parameters"=variant}) -> ()  [unwired: 2 in, 3 out]
      }
      event "Telescope Type": Value Change {
        n229 = event-data() -> ("CtlRef"=w434:refnum<vi>)  [unwired: 1 in, 5 out]
        n230 = property class="Ring (strict)"(reference=w434) -> ("Strings []"=w433:string[])  [unwired: 1 in, 2 out]
        n231 = Unbundle By Name(w430) -> ("state"=w429:refnum<user-event>)
        n232 = Generate User Event(user event=w429, event data cluster="Reinit" ("event data")) -> ()  [unwired: 2 in, 2 out]
        n233 = Index Array(array=w433, index="Telescope Type") -> (element=w426:string)
        n234 = call "CC Set Device By Name.vi"("Device Name"=w426, "Device Type"="Telescope") -> ()  [unwired: 8 in, 2 out]
        n235 = Bundle By Name(cluster=w430, "Telescope Name"=w426) -> (w431:T17)
      }
      event "Reconnect": Value Change {
        n236 = event-data() -> ()  [unwired: 1 in, 6 out]
        n237 = Unbundle By Name(w437) -> ("state"=w436:refnum<user-event>)
        n238 = Generate User Event(user event=w436, event data cluster="Reinit" ("event data")) -> ()  [unwired: 2 in, 2 out]
      }
      event Value Change {
        n239 = event-data() -> ()  [unwired: 1 in, 6 out]
        n240 = case shown="\"User\", Default" "Mode" {
          tunnel: [bool[] [TRUE, FALSE, FALSE] bool[] [TRUE, TRUE, TRUE]] -> w438
          frame "User", Default {
          }
          frame "Engineering" {
          }
        }
        n241 = property on="Tab Control" class="TabCtl (strict)"() -> ("Pages"=w439:refnum<vi>[])  [unwired: 2 in, 2 out]
        n242 = for {
          tunnel: w439 -> [w443] mode=indexing
          tunnel: w438 -> [w442] mode=indexing
          n243 = property class="Page"(reference=w443, "PageVis"=w442) -> ()  [unwired: 1 in, 2 out]
        }
      }
      event "Close": Value Change {
        n244 = event-data() -> ()  [unwired: 1 in, 2 out]
        n245 = Unbundle By Name(w448) -> ("state"=w447:refnum<user-event>)
        n246 = Generate User Event(user event=w447, event data cluster="Shutdown" ("event data")) -> ()  [unwired: 2 in, 2 out]
      }
    }
  }
  n247 = flat-sequence {
    tunnel: w1 -> [_]
    frame #0 {
      n248 = property class="App"() -> ("App.Kind"=w450:T26)  [unwired: 2 in, 2 out]
      n249 = Equal?(x=w450, y=T26."Run Time System" ("Application:Kind")) -> (x = y?=w449:bool)
      n250 = Quit LabVIEW(quit? (T)=w449) -> ()
    }
  }
